vi "Unnest-Macro.vi"(7 "expand":bool=TRUE, 8 "Sequences folder path":path=path "C:/Users/shared/Sequences", 9 "Use absolute sequence path":bool, 10 "platform":u16(ring) items=["Mac", "PC"], 11 "Item Names IN":string[](array[string])=["Wait for 11 s", "Run Macro C:\\Users\\shared\\NML Data Acquisition\\monovu\\sub1.txt", "Wait for 131 s", "Run Macro C:\\Users\\shared\\NML Data Acquisition\\monovu\\sub2.txt", "Wait for 131 s", "END SEQUENCE"]) -> (2 "unnested items":string[](array[string])=["Wait for 11 s", "Wait for 2.1 s", "Wait for 2.2 s", "Wait for 2.3 s", "Wait for 3 s", "----------    end of sequence line removed", "----------    end of sequence line removed", "----------    end of sequence line removed", "----------    end of sequence line removed", "END SUBsequence", "Wait for 131 s", "Wait for 2.2 s", "Wait for 2.3 s", "Wait for 3 s", "----------    end of sequence line removed", "----------    end of sequence line removed", "----------    end of sequence line removed", "END SUBsequence", "Wait for 131 s", "END SEQUENCE"], 3 "item index":string[](array[string])=["0.0", "1.0", "1.1", "1.2", "1.3", "1.4", "1.5", "1.6", "1.7", "1.8", "2.0", "3.0", "3.1", "3.2", "3.3", "3.4", "3.5", "3.6", "4.0", "5.0"])   [LabVIEW 2025]
uses:
  <vilib>/Utility/error.llb/Trim Whitespace One-Sided.vi
panel:
  # "(if abs. path not used)"
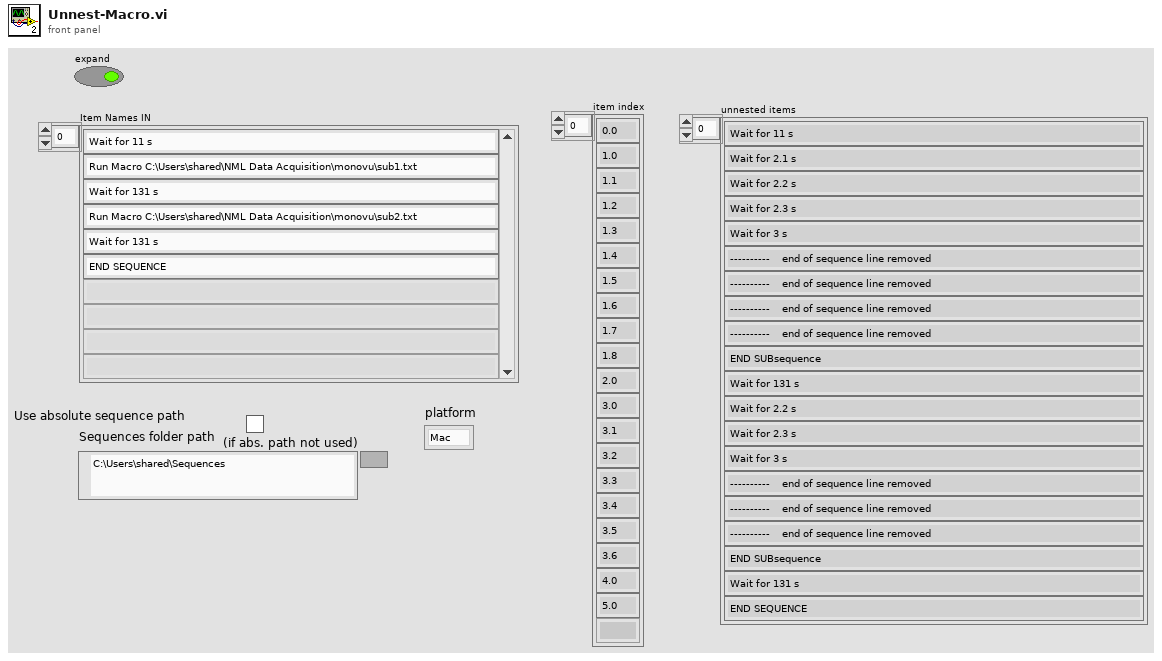
[diagram p1: front panel]
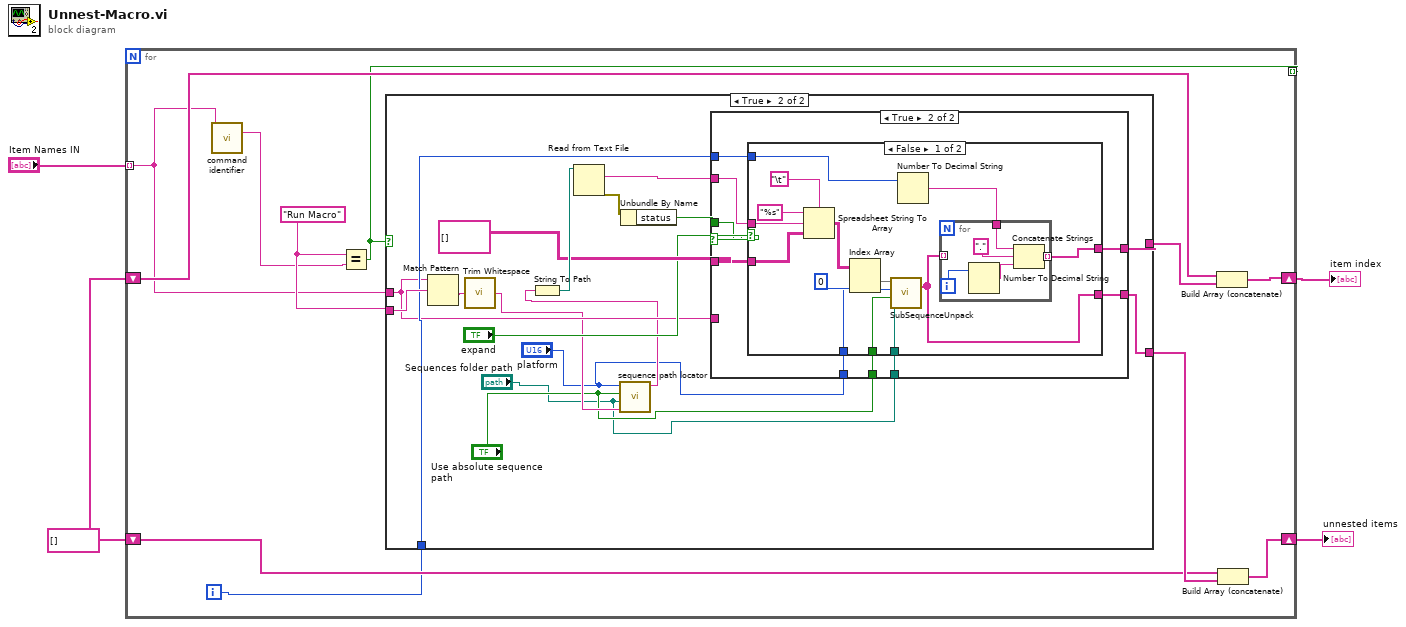
[diagram p0: block diagram]
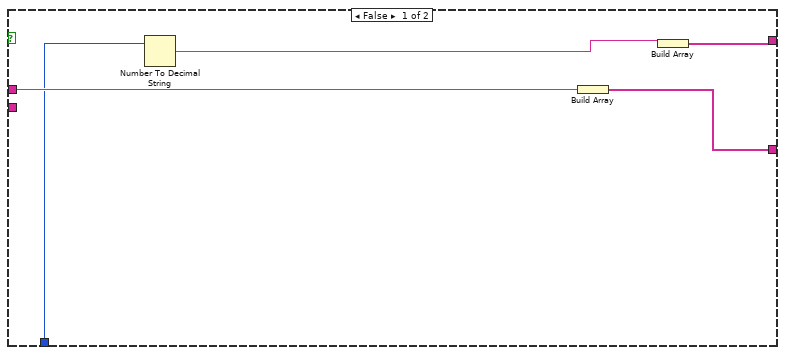
[diagram p2: hidden frame]
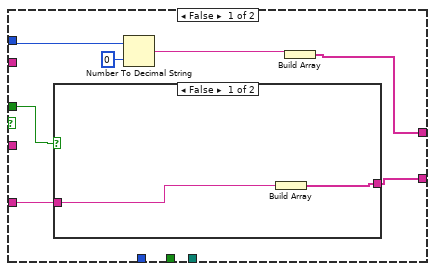
[diagram p3: hidden frame]
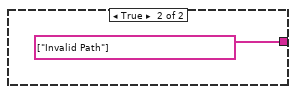
[diagram p4: hidden frame]
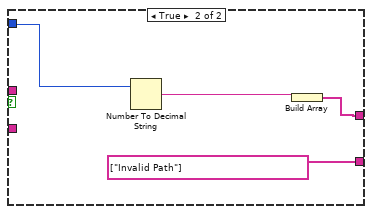
[diagram p5: hidden frame]
diagram:
  w3 = string[] []
  n1 = for {
    tunnel: "Item Names IN" -> [w6] mode=indexing
    shift-right: [w13] -> w1
    shift-left: w3 -> [w12]
    shift-right: [w9] -> w2
    shift-left: w3 -> [w8]
    tunnel: [w7] -> _ mode=indexing
    i -> [w11]
    w15 = "Run Macro" ("y")
    n2 = call "command identifier.vi"("Input command"=w6) -> ("Identifield command"=w5:string)  [unwired: 10 in]
    n3 = Equal?(x=w15, y=w5) -> (x = y?=w7:bool)
    n4 = case shown="True" w7 {
      tunnel: w15 -> [_ w37]
      tunnel: w6 -> [w20 w26]
      tunnel: [w19 w34] -> w14
      tunnel: w11 -> [w18 w35]
      tunnel: [w17 w33] -> w10
      frame False {
        n5 = Number To Decimal String(number=w18) -> (decimal integer string=w16:string)  [unwired: 1 in]
        n6 = Build Array(w20) -> (w19:string[])
        n7 = Build Array(w16) -> (w17:string[])
      }
      frame True {
        n8 = Match Pattern(string=w26, regular expression=w37) -> (after substring=w36:string)  [unwired: 1 in, 3 out]
        n9 = call <vilib>:"Trim Whitespace.vi"("string"=w36) -> ("trimmed string"=w25:string)  [unwired: 1 in]
        n10 = call "sequence path locator.vi"("sequence path"=w25, "Sequences folder path"="Sequences folder path", "Use absolute sequence path"="Use absolute sequence path", "platform"="platform") -> ("modified path"=w24:string)  [unwired: 7 in]
        n11 = String To Path(string=w24) -> (path=w32:path)
        n12 = Read from Text File(file (use dialog)=w32) -> (text=w31:string, error out=w29:errorcluster)  [unwired: 3 in, 2 out]
        n13 = Unbundle By Name(w29) -> ("status"=w28:bool)
        n14 = case shown="True" "expand" {
          tunnel: w35 -> [w41 w56]
          tunnel: [w44 w55] -> w34
          tunnel: [w40 w54] -> w33
          tunnel: w31 -> [_ w53]
          tunnel: string[][] [] -> [_ w52]
          tunnel: w28 -> [w43 w51]
          tunnel: w26 -> [w39 _]
          tunnel: "platform" -> [_ w50]
          tunnel: "Use absolute sequence path" -> [_ w49]
          tunnel: "Sequences folder path" -> [_ w48]
          frame False {
            n15 = case shown="False" w43 {
              tunnel: [w45 string[] ["Invalid Path"] ("output sequences")] -> w44
              tunnel: w39 -> [w46 _]
              frame False {
                n16 = Build Array(w46) -> (w45:string[])
              }
              frame True {
              }
            }
            n17 = Number To Decimal String(number=w41, width (-)=i16 0) -> (decimal integer string=w42:string)
            n18 = Build Array(w42) -> (w40:string[])
          }
          frame True {
            n19 = case shown="False" w51 {
              tunnel: w56 -> [w70 w79]
              tunnel: [w68 string[] ["Invalid Path"] ("output sequences")] -> w55
              tunnel: [w67 w78] -> w54
              tunnel: w53 -> [w66 _]
              tunnel: w52 -> [w62 _]
              tunnel: w50 -> [w59 _]
              tunnel: w49 -> [w58 _]
              tunnel: w48 -> [w57 _]
              frame False {
                n20 = Spreadsheet String To Array(delimiter (Tab)="\t", format string="%s", spreadsheet string=w66, array type (2D Dbl)=w62) -> (array=w63:string[][])
                n21 = Index Array(array=w63, index (col)=0 ("index (row)")) -> (element=w61:string[])  [unwired: 1 in]
                n22 = call "SubSequenceUnpack.vi"("Sequences folder path"=w57, "Use absolute sequence path"=w58, "platform"=w59, "input sequences"=w61) -> ("output sequences"=w68:string[])  [unwired: 7 in]
                n23 = Number To Decimal String(number=w70) -> (decimal integer string=w69:string)  [unwired: 1 in]
                n24 = for {
                  tunnel: w68 -> [_] mode=indexing
                  tunnel: w69 -> [w72]
                  tunnel: [w71] -> w67 mode=indexing
                  i -> [w74]
                  n25 = Number To Decimal String(number=w74) -> (decimal integer string=w73:string)  [unwired: 1 in]
                  n26 = Concatenate Strings(w72, "." ("string"), w73) -> (w71:string)
                }
              }
              frame True {
                n27 = Number To Decimal String(number=w79) -> (decimal integer string=w76:string)  [unwired: 1 in]
                n28 = Build Array(w76) -> (w78:string[])
              }
            }
          }
        }
      }
    }
    n29 = Build Array (concatenate)(w8, w10) -> (w9:string[])
    n30 = Build Array (concatenate)(w12, w14) -> (w13:string[])
  }
  "item index" <- w2
  "unnested items" <- w1
